vi "ID.vi"(8 "error in (no error)":errorcluster, 11 "Response in":refnum<class "Response.lvclass">) -> (0 "error out":errorcluster, 2 "ID":string, 3 "Response out":refnum<class "Response.lvclass">)   [LabVIEW 2022 SP3, in "obs-websocket-lv.lvlib" / "Response.lvclass"]
uses:
  Response.lvclass
  Response.lvclass/Response.ctl
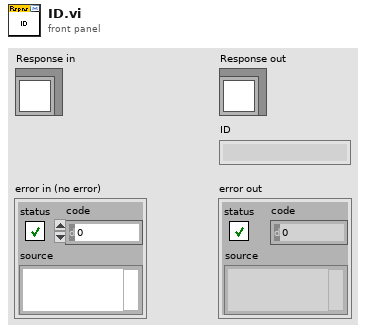
[diagram p1: front panel]
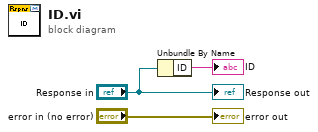
[diagram p0: block diagram]
diagram:
  n1 = Unbundle By Name("Response in") -> ("ID"=→"ID":string)
  "error out" <- "error in (no error)"
  "Response out" <- "Response in"
